vi "Get Configuration Cluster.vi"(8 "error in (no error)":errorcluster, 11 "Group Configuration in":refnum<class "Group Configuration.lvclass">) -> (0 "error out":errorcluster, 2 "group configuration":T1={"core"={"name"="Group", "direction"=enum."Tx", "cycle timing"={"priority"=100, "decimation"=1, "offset"=0}, "timeout behavior"=enum."Increment Late Count", "enable conversion"=FALSE}, "component settings"=[], "transfers"=[]} {"transfers"."channels"."core"."string offset" format="%d bytes"}, 3 "Group Configuration out":refnum<class "Group Configuration.lvclass">)   [LabVIEW 2021, in "DSF Core.lvlib" / "Group Configuration.lvclass"]
uses:
  Group Configuration.lvclass
  C:/dev/git/custom-devices/niveristand-data-sharing-framework-custom-device/Source/Core/Classes/Configuration/Core/Core Configuration.lvclass
  Typedefs/DSF Engine Transfer Group Configuration.ctl
  Typedefs/Core Group Configuration.ctl
  Typedefs/DSF Direction.ctl
  Typedefs/DSF Timing Info.ctl
  Typedefs/DSF Timeout Behavior.ctl
  Typedefs/DSF Settings Info.ctl
  Typedefs/DSF Engine Transfer Configuration.ctl
  Typedefs/Core Transfer Configuration.ctl
  Typedefs/DSF Engine Channel Configuration.ctl
  Typedefs/Core Channel Configuration.ctl
  Typedefs/DSF Data Type.ctl
  Group Configuration.lvclass/Group Configuration.ctl
  Transfer/Transfer Configuration.lvclass
  DSF Core.lvlib
  Core Configuration.lvclass
  Channel/Channel Configuration.lvclass
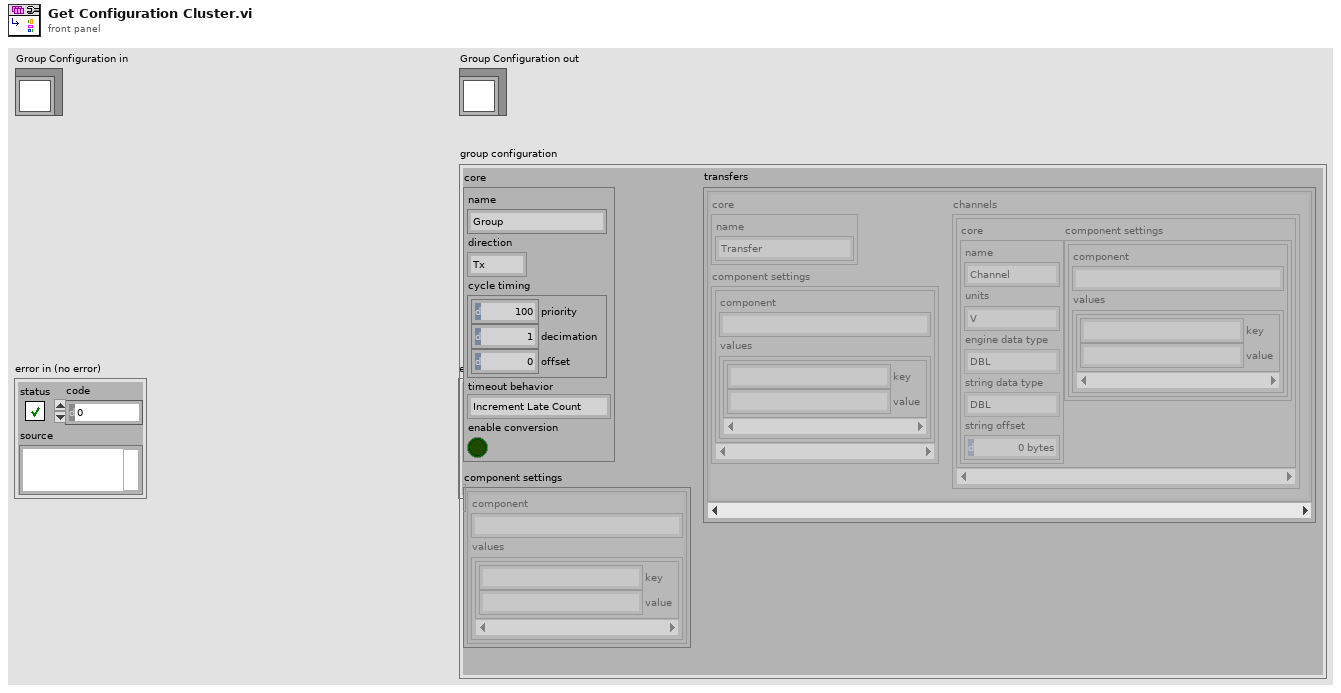
[diagram p1: front panel]
types:
  T1 = typedef "DSF Core.lvlib/DSF Engine Transfer Group Configuration.ctl" = cluster{"core":T2, "component settings":T6[], "transfers":T7[]}
  T2 = typedef "DSF Core.lvlib/Group Configuration.lvclass/Core Group Configuration.ctl" = cluster{"name":string, "direction":T3, "cycle timing":T4, "timeout behavior":T5, "enable conversion":bool}
  T3 = typedef "DSF Core.lvlib/DSF Direction.ctl" = enum8{"Tx", "Rx"}
  T4 = typedef "DSF Core.lvlib/DSF Timing Info.ctl" = cluster{"priority":u64, "decimation":u64, "offset":u64}
  T5 = typedef "DSF Core.lvlib/DSF Timeout Behavior.ctl" = enum8{"Increment Late Count", "Throw Error"}
  T6 = typedef "DSF Core.lvlib/DSF Settings Info.ctl" = cluster{"component":string, "values":cluster{"key":string, "value":string}[]}
  T7 = typedef "DSF Core.lvlib/DSF Engine Transfer Configuration.ctl" = cluster{"core":T8, "component settings":T6[], "channels":T9[]}
  T8 = typedef "DSF Core.lvlib/Transfer Configuration.lvclass/Core Transfer Configuration.ctl" = cluster{"name":string}
  T9 = typedef "DSF Core.lvlib/DSF Engine Channel Configuration.ctl" = cluster{"core":T10, "component settings":T6[]}
  T10 = typedef "DSF Core.lvlib/Channel Configuration.lvclass/Core Channel Configuration.ctl" = cluster{"name":string, "units":string, "engine data type":T11, "string data type":T11, "string offset":u64}
  T11 = typedef "DSF Core.lvlib/DSF Data Type.ctl" = enum8{"Bool", "SGL", "DBL", "I8", "I16", "I32", "I64", "U8", "U16", "U32", "U64"}
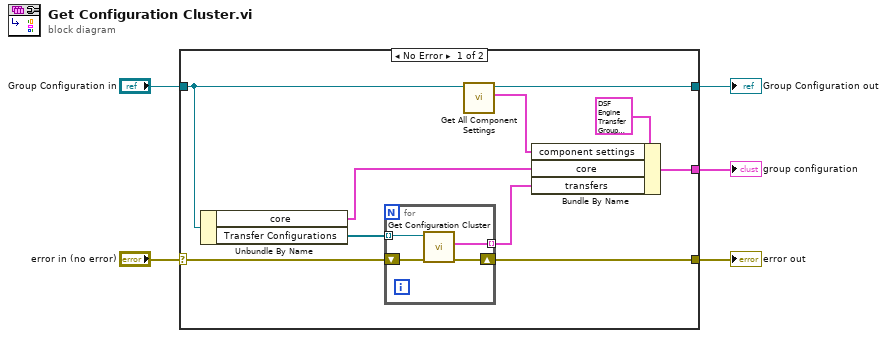
[diagram p0: block diagram]
diagram:
  n1 = case shown="No Error" "error in (no error)" {
    selector: "error in (no error)" -> [w15 w21]
    tunnel: [w14 w21] -> w4
    tunnel: [w8 w20] -> w2
    tunnel: "Group Configuration in" -> [w7 w20]
    tunnel: [w10 _] -> w1
    frame No Error {
      n2 = Unbundle By Name(w7) -> ("core"=w6:T2, "Transfer Configurations"=w13:refnum<class "Transfer Configuration.lvclass">[])
      n3 = for {
        shift-right: [w18] -> w14
        shift-left: w15 -> [w19]
        tunnel: w13 -> [w17] mode=indexing
        tunnel: [w16] -> w11 mode=indexing
        n4 = call "Get Configuration Cluster.vi"("error in (no error)"=w19, "Transfer Configuration in"=w17) -> ("error out"=w18:errorcluster, "transfer configuration"=w16:T7)  [unwired: 7 in, 1 out]
      }
      n5 = call "Get All Component Settings.vi"("Runtime Configuration in"=w7) -> ("component settings"=w9:T6[], "Runtime Configuration out"=w8:refnum<class "Group Configuration.lvclass">)  [unwired: 8 in, 1 out]
      n6 = Bundle By Name(cluster=T1 {"core"={"name"="Group", "direction"=enum."Tx", "cycle timing"={"priority"=100, "decimation"=1, "offset"=0}, "timeout behavior"=enum."Increment Late Count", "enable conversion"=FALSE}, "component settings"=[], "transfers"=[]} ("group configuration"), "component settings"=w9, "core"=w6, "transfers"=w11) -> (w10:T1)
    }
    frame Error {
    }
  }
  "error out" <- w4
  "Group Configuration out" <- w2
  "group configuration" <- w1
